vi "Test2.vi"() -> ()   [LabVIEW 2013]
panel:
  in  "InitCode":string="u[0]=0;\nu[1]=0;"
  out "controlState":dbl[](array[numeric])=[-6.74]
  in  "Code":string="x=plantState[1];\nu[0]=-x;\nfor (i=0; i<1000000 ; i++);"
  in  "plantState":dbl[](array[numeric])=[1.0, 6.74]
  out "evals1":i32=713
  out "T1":u32(graph)=320
  in  "stop":bool=TRUE
  out "error out":errorcluster
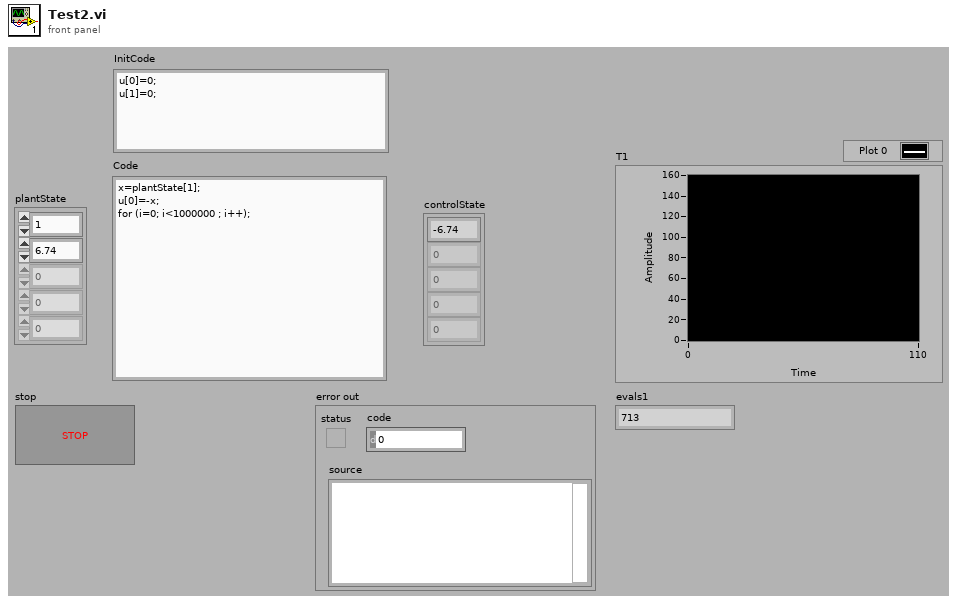
[diagram p1: front panel]
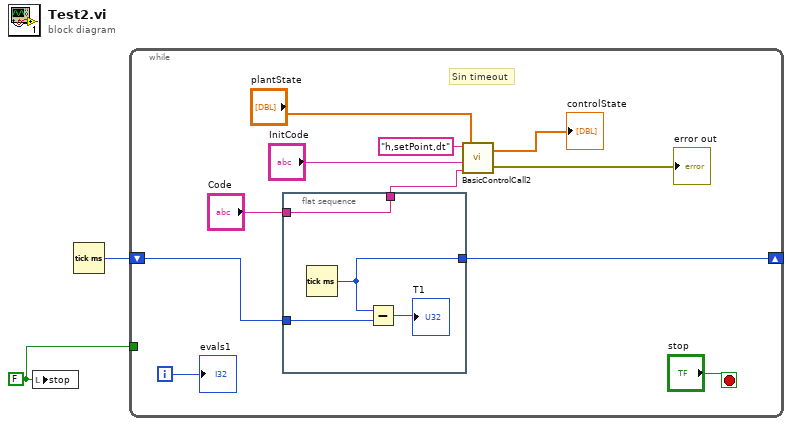
[diagram p0: block diagram]
diagram:
  w2 = FALSE ("stop")
  n1 = local write "stop"(w2) -> ()
  n2 = Tick Count (ms)() -> (millisecond timer value=w1:u32)
  n3 = while {
    shift-right: [w9] -> _
    shift-left: w1 -> [w8]
    tunnel: w2 -> [_]
    i -> [w12]
    stop <- "stop" stop-if-true
    # "Sin timeout"
    n4 = flat-sequence {
      tunnel: [w17] -> w9
      tunnel: w8 -> [w16]
      tunnel: [w14] -> w6
      tunnel: "Code" -> [w14]
      frame #0 {
        n5 = Tick Count (ms)() -> (millisecond timer value=w17:u32)
        n6 = Subtract(x=w17, y=w16) -> (x-y=→"T1":u32)
      }
    }
    n7 = call "BasicControlCall2.vi"("Code"=w6, "InitCode"="InitCode", "plantState"="plantState", "variablesIN"="h,setPoint,dt") -> ("error"=→"error out":errorcluster, "controlState"=→"controlState":dbl[])
    "evals1" <- w12
  }
